vi "PNG WriteFileWithAlpha.vi"(8 "error in (no error)":errorcluster, 10 "image data":T1, 11 "Path to write (dialog)":path) -> (0 "error out":errorcluster, 3 "Selected Path":path)   [LabVIEW 2017]
uses:
  <vilib>/picture/picture.llb/imagedata.ctl
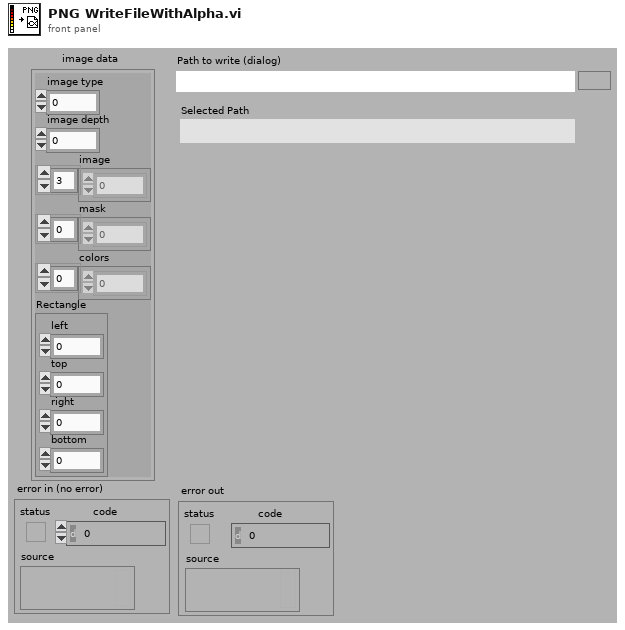
[diagram p1: front panel]
types:
  T1 = typedef "imagedata.ctl" = cluster{"image type":i32, "image depth":i32, "image":u8[], "mask":u8[], "colors":u32[], "Rectangle":cluster{"left":i16, "top":i16, "right":i16, "bottom":i16}}
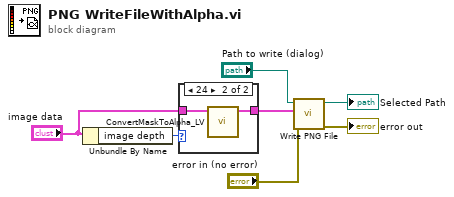
[diagram p0: block diagram]
diagram:
  n1 = Unbundle By Name("image data") -> ("image depth"=w7:i32)
  n2 = case shown="24" w7 {
    tunnel: "image data" -> [w8 w10]
    tunnel: [w8 w9] -> w5
    frame 0, Default {
    }
    frame 24 {
      n3 = call "ConvertMaskToAlpha_LV.vi"("image data"=w10) -> ("image data out"=w9:T1)  [unwired: 10 in]
    }
  }
  n4 = call <vilib>:"Write PNG File.vi"("error in (no error)"="error in (no error)", "image data"=w5, "path to PNG file"="Path to write (dialog)") -> ("error out"=→"error out":errorcluster, "path"=→"Selected Path":path)  [unwired: 7 in]
